vi "Set Attribute.vi"(4 "Attribute [\"Info\"]":string="Info", 5 "Overwrite? [T]":bool=TRUE, 6 "Text":string, 7 "Error [Last]":enum16{"First", "Last", "All"}(ring)=enum."Last", 10 "error in (no error)":errorcluster) -> (2 "error out":errorcluster)   [LabVIEW 2020, in "Multiple Errors.lvclass"]
uses:
  Multiple Errors.lvclass
  <vilib>/MultiError/TokenizeJSON/Multi Error Cluster.lvlib
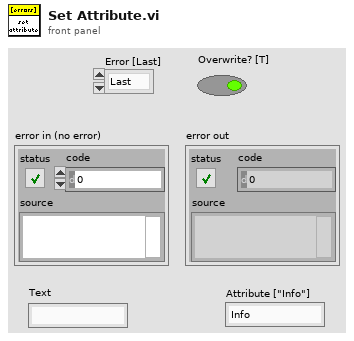
[diagram p1: front panel]
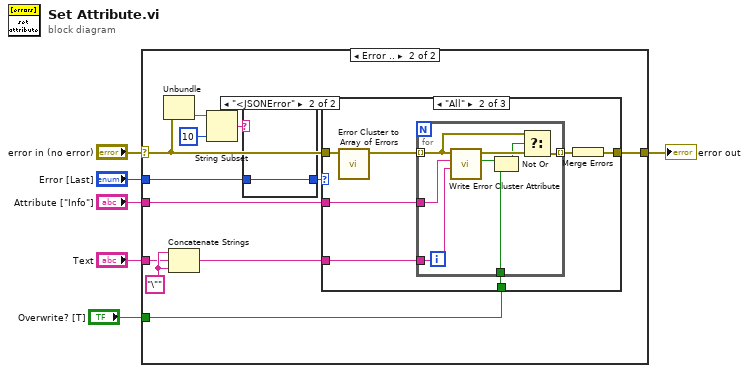
[diagram p0: block diagram]
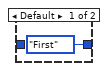
[diagram p3: hidden frame]
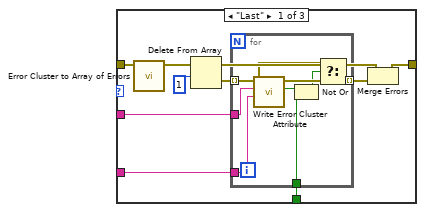
[diagram p4: hidden frame]
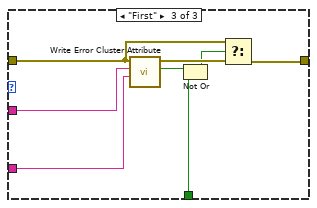
[diagram p5: hidden frame]
diagram:
  n1 = case shown="Error .." "error in (no error)" {
    selector: "error in (no error)" -> [w7 w10]
    tunnel: "Attribute [\"Info\"]" -> [_ w15]
    tunnel: [w7 w19] -> w5
    tunnel: "Text" -> [_ w17]
    tunnel: "Error [Last]" -> [_ w13]
    tunnel: "Overwrite? [T]" -> [_ w8]
    frame No Error {
    }
    frame Error {
      w18 = "\"" ("string")
      n2 = Unbundle(w10) -> ("source"=w9:string)  [unwired: 2 out]
      n3 = Concatenate Strings(w18, w17, w18) -> (w16:string)
      n4 = String Subset(string=w9, length (rest)=10 ("length (rest)")) -> (substring=w11:string)  [unwired: 1 in]
      n5 = case shown="\"<JSONError\"" w11 {
        tunnel: w13 -> [_ w21]
        tunnel: [enum16{"First", "Last", "All"}."First" ("Error [Last]") w21] -> w12
        frame Default {
        }
        frame "<JSONError" {
        }
      }
      n6 = case shown="\"All\"" w12 {
        tunnel: w15 -> [w31 w46 w62]
        tunnel: [w30 w45 w58] -> w19
        tunnel: w16 -> [w29 w44 w61]
        tunnel: w10 -> [w28 w43 w59]
        tunnel: w8 -> [w22 w40 w55]
        frame "Last" {
          n7 = call <vilib>:"Error Cluster to Array of Errors.vi"("error"=w28) -> ("array of errors"=w27:errorcluster[])  [unwired: 10 in]
          n8 = Delete From Array(array=w27, length=1) -> (deleted portion=w24:errorcluster[], array with subset deleted=w23:errorcluster[])  [unwired: 1 in]
          n9 = for {
            tunnel: [w36] -> w26 mode=indexing
            tunnel: w31 -> [w39]
            tunnel: w24 -> [w35] mode=indexing
            tunnel: w29 -> [w38]
            tunnel: w22 -> [w32]
            n10 = call <vilib>:"Write Error Cluster Attribute.vi"("JSON value"=w38, "attribute name"=w39, "error in"=w35) -> ("created?"=w34:bool, "error out"=w37:errorcluster)  [unwired: 7 in]
            n11 = Not Or(1:w32, 2:w34) -> (0:w33:bool)
            n12 = Select(t=w35, s=w33, f=w37) -> (s? t:f=w36:errorcluster)
          }
          n13 = Merge Errors(w23, w26) -> (w30:errorcluster)
        }
        frame "All" {
          n14 = call <vilib>:"Error Cluster to Array of Errors.vi"("error"=w43) -> ("array of errors"=w42:errorcluster[])  [unwired: 10 in]
          n15 = for {
            tunnel: [w50] -> w41 mode=indexing
            tunnel: w46 -> [w54]
            tunnel: w42 -> [w51] mode=indexing
            tunnel: w44 -> [w53]
            tunnel: w40 -> [w48]
            n16 = call <vilib>:"Write Error Cluster Attribute.vi"("JSON value"=w53, "attribute name"=w54, "error in"=w51) -> ("created?"=w49:bool, "error out"=w52:errorcluster)  [unwired: 7 in]
            n17 = Not Or(1:w48, 2:w49) -> (0:w47:bool)
            n18 = Select(t=w51, s=w47, f=w52) -> (s? t:f=w50:errorcluster)
          }
          n19 = Merge Errors(w41) -> (w45:errorcluster)
        }
        frame "First" {
          n20 = call <vilib>:"Write Error Cluster Attribute.vi"("JSON value"=w61, "attribute name"=w62, "error in"=w59) -> ("created?"=w57:bool, "error out"=w60:errorcluster)  [unwired: 7 in]
          n21 = Not Or(1:w55, 2:w57) -> (0:w56:bool)
          n22 = Select(t=w59, s=w56, f=w60) -> (s? t:f=w58:errorcluster)
        }
      }
    }
  }
  "error out" <- w5
